vi "main GUI Caller.vi"() -> ()   [LabVIEW 2015]
panel:
  in  "stop":bool
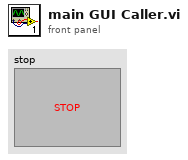
[diagram p1: front panel]
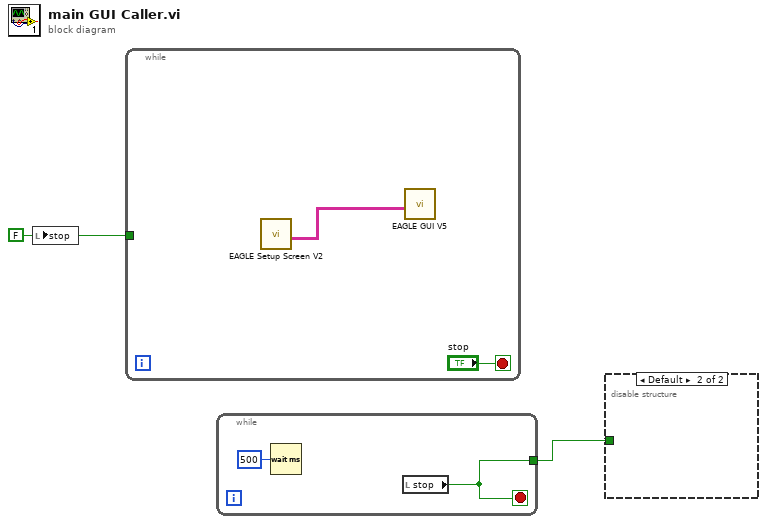
[diagram p0: block diagram]
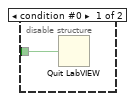
[diagram p2: hidden frame]
diagram:
  w2 = FALSE ("stop")
  n1 = local write "stop"(w2) -> ()
  n2 = while {
    tunnel: w2 -> [_]
    stop <- "stop" stop-if-true
    n3 = call "EAGLE Setup Screen V2.vi"() -> ("Table Control"=w3:string[][])  [unwired: 11 in]
    n4 = call "EAGLE GUI V5.vi"("TableIn"=w3) -> ()  [unwired: 11 in]
  }
  n5 = while {
    tunnel: [w6] -> w1
    stop <- w6 stop-if-true
    n6 = Wait (ms)(milliseconds to wait=u32 500) -> ()  [unwired: 1 out]
    n7 = local read "stop"() -> (w6:bool)
  }
  n8 = disable-structure shown="Default" {
    disable-tunnel: w1 -> [w7 _]
    frame condition #0 {
      n9 = Quit LabVIEW(quit? (T)=w7) -> ()
    }
    frame condition #1 (active) {
    }
  }
